vi "read_console_stream.vi"(8 "error in (no error)":errorcluster, 11 "console.provider in":refnum<class "console.provider.lvclass">) -> (0 "error out":errorcluster, 1 "abort":bool, 2 "log":T1 {"datetime" format="%<%x %.3X>T"}, 3 "console.provider out":refnum<class "console.provider.lvclass">)   [LabVIEW 2021, in "console.provider.lvclass"]
uses:
  console.provider.lvclass
  system.logging/log_entry.ctl
  system.logging/severity.ctl
  console.provider.lvclass/console.provider.ctl
  system.logging/system.logging.lvclass
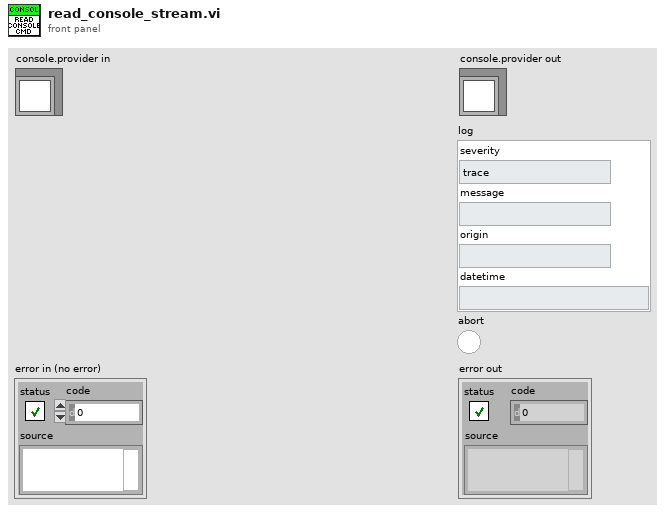
[diagram p1: front panel]
types:
  T1 = typedef "system.logging.lvclass/log_entry.ctl" = cluster{"severity":T2, "message":string, "origin":string, "datetime":timestamp}
  T2 = typedef "system.logging.lvclass/severity.ctl" = enum8{"trace", "debug", "info", "warning", "error"}
  T3 = typedef "console.provider.lvclass/console_payload.ctl" = cluster{"console_cmd":T4, "log":T1}
  T4 = typedef "console.provider.lvclass/console_commands.ctl" = enum16{"close", "print"}
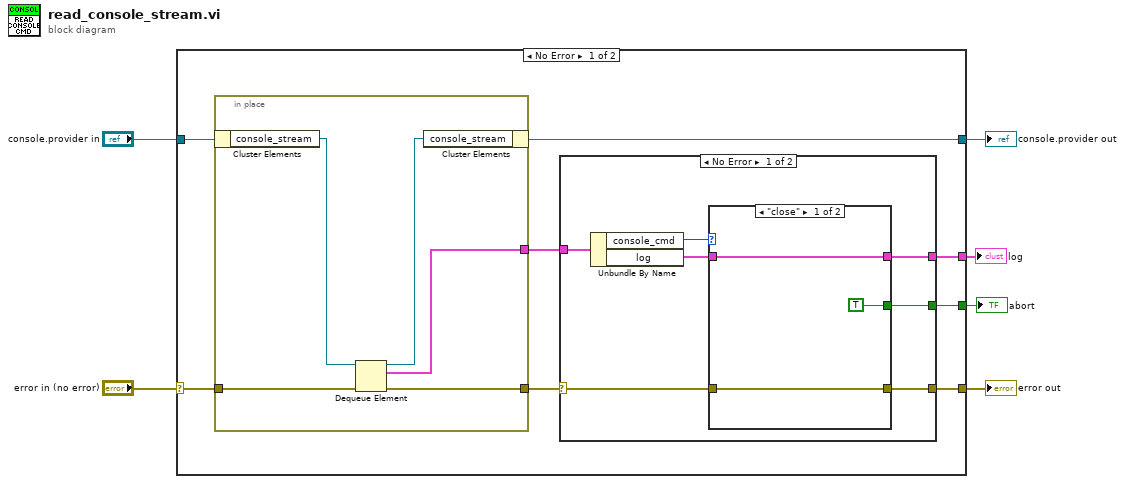
[diagram p0: block diagram]
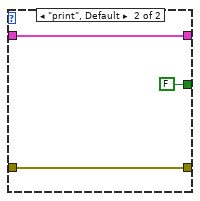
[diagram p2: hidden frame]
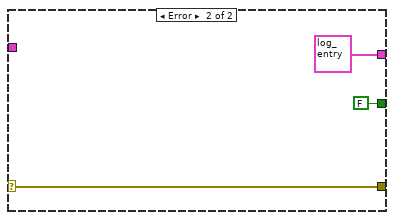
[diagram p3: hidden frame]
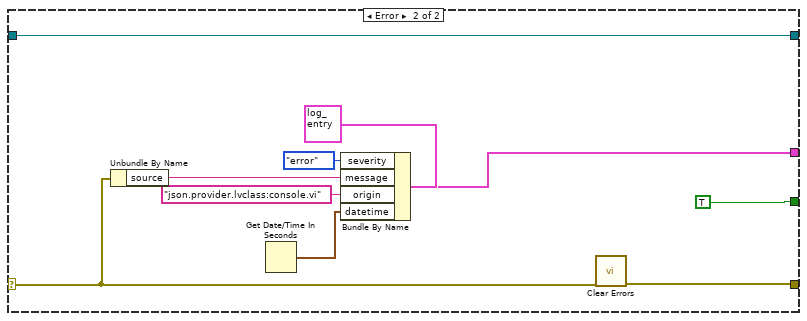
[diagram p4: hidden frame]
diagram:
  n1 = case shown="No Error" "error in (no error)" {
    selector: "error in (no error)" -> [w13 w40]
    tunnel: [w9 w41] -> w5
    tunnel: [w12 w45] -> w3
    tunnel: "console.provider in" -> [w14 w45]
    tunnel: [w10 w37] -> w2
    tunnel: [w8 TRUE] -> w1
    frame No Error {
      n2 = in-place {
        in-place-border: w13 -> [w35]
        in-place-border: [w31] -> w11
        in-place-border: [w32] -> w7
        n3 = in-place-cluster #1(w14) -> ("console_stream"=w34:refnum<queue>)
        n4 = Dequeue Element(queue=w34, error in (no error)=w35) -> (queue out=w33:refnum<queue>, element=w31:T3, error out=w32:errorcluster)  [unwired: 1 in, 1 out]
        n5 = in-place-cluster #1("console_stream"=w33) -> (w12:refnum<class "console.provider.lvclass">)
      }
      n6 = case shown="No Error" w7 {
        selector: w7 -> [w15 w29]
        tunnel: w11 -> [w21 _]
        tunnel: [w18 T1 {"severity"=enum."trace", "message"="", "origin"="", "datetime"=timestamp(0 s since 1904-01-01)} ("log")] -> w10
        tunnel: [w17 w29] -> w9
        tunnel: [w16 FALSE] -> w8
        frame No Error {
          n7 = Unbundle By Name(w21) -> ("console_cmd"=w20:T4, "log"=w19:T1)
          n8 = case shown="\"close\"" w20 {
            tunnel: w19 -> [w24 w27]
            tunnel: [w24 w27] -> w18
            tunnel: w15 -> [w23 w25]
            tunnel: [w23 w25] -> w17
            tunnel: [TRUE FALSE] -> w16
            frame "close" {
            }
            frame "print", Default {
            }
          }
        }
        frame Error {
        }
      }
    }
    frame Error {
      n9 = Unbundle By Name(w40) -> ("source"=w39:string)
      n10 = Get Date/Time In Seconds() -> (seconds since 1Jan1904=w42:timestamp)
      n11 = Bundle By Name(cluster=T1 {"severity"=enum."error", "message"="", "origin"="", "datetime"=timestamp(0 s since 1904-01-01)} ("log"), "severity"=severity."error", "message"=w39, "origin"="json.provider.lvclass:console.vi", "datetime"=w42) -> (w37:T1)
      n12 = call <vilib>:"Clear Errors.vi"("error in (no error)"=w40) -> ("error out"=w41:errorcluster)  [unwired: 5 in, 1 out]
    }
  }
  "error out" <- w5
  "console.provider out" <- w3
  "log" <- w2
  "abort" <- w1
